vi "exp1_虚拟温度计.vi"() -> ()   [LabVIEW 2021]
panel:
  out "华氏度":dbl(knob) scale=0.0..200.0
  out "数据记录":string[](array[string])
  in  "停止按钮":bool
  out "温度模式":bool
  in  "开关":bool
  in  "模式":bool
  out "温度":dbl
  out "温度计":dbl(slide) scale=250.0..400.0
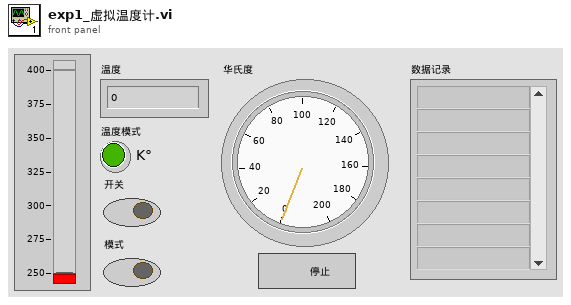
[diagram p1: front panel]
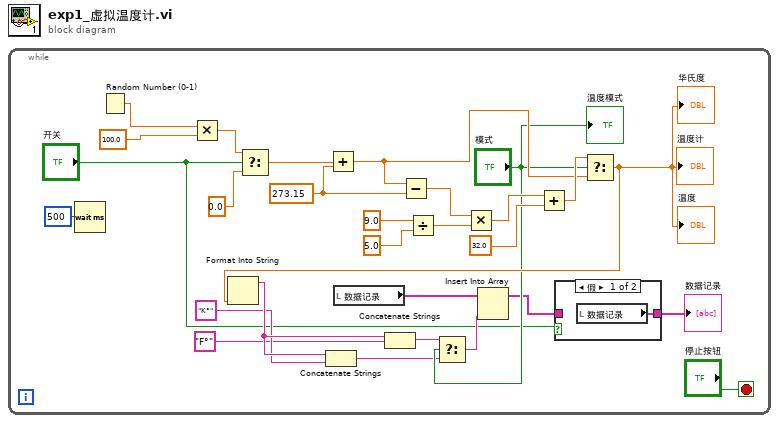
[diagram p0: block diagram]
diagram:
  n1 = while {
    stop <- "停止按钮" stop-if-true
    w23 = 273.15
    n2 = Wait (ms)(milliseconds to wait=500) -> ()  [unwired: 1 out]
    n3 = Random Number (0-1)() -> (number: 0 to 1=w17:dbl)
    n4 = Multiply(x=w17, y=100.0) -> (x*y=w15:dbl)
    n5 = Select(t=w15, s="开关", f=0.0) -> (s? t:f=w25:dbl)
    n6 = Add(x=w25, y=w23) -> (x+y=w13:dbl)
    n7 = local read "数据记录"() -> (w10:string[])
    n8 = Subtract(x=w13, y=w23) -> (x-y=w20:dbl)
    n9 = Divide(x=9.0, y=5.0) -> (x/y=w19:dbl)
    n10 = Multiply(x=w20, y=w19) -> (x*y=w18:dbl)
    n11 = Add(x=w18, y=32.0) -> (x+y=w14:dbl)
    n12 = Select(t=w14, s="模式", f=w13) -> (s? t:f=w12:dbl)
    "温度计" <- w12
    "温度" <- w12
    "华氏度" <- w12
    n13 = Format Into String(w12) -> (resulting string=w9:string)  [unwired: 3 in, 1 out]
    n14 = Concatenate Strings(w9, "K°") -> (w7:string)
    n15 = Concatenate Strings(w9, "F°") -> (w6:string)
    n16 = Select(t=w6, s="模式", f=w7) -> (s? t:f=w8:string)
    n17 = Insert Into Array(array=w10, new element=w8) -> (w2:string[])  [unwired: 1 in]
    n18 = case shown="假" "开关" {
      tunnel: [w29 w30] -> w3
      tunnel: w2 -> [_ w30]
      frame False {
        n19 = local read "数据记录"() -> (w29:string[])
      }
      frame True {
      }
    }
    "数据记录" <- w3
    "温度模式" <- "模式"
  }
